vi "Add Numbers.vi"(8 "error in (no error)":errorcluster, 9 "Number 2":dbl, 10 "Number 1":dbl, 11 "Addition Actor in":refnum<class "Addition Actor.lvclass">) -> (0 "error out":errorcluster, 3 "Addition Actor out":refnum<class "Addition Actor.lvclass">)   [LabVIEW 2024, in "Addition Actor.lvclass"]
uses:
  Addition Actor.lvclass
  C:/Program Files/National Instruments/LabVIEW 2024/vi.lib/ActorFramework/Actor/Actor.lvclass
  <vilib>/ActorFramework/Actor/Actor.lvclass/Actor.ctl
  <vilib>/ActorFramework/Actor/Actor.lvclass
  Calculator Actor/Calculator Actor Messages/Addition Result Msg/Addition Result Msg.lvclass
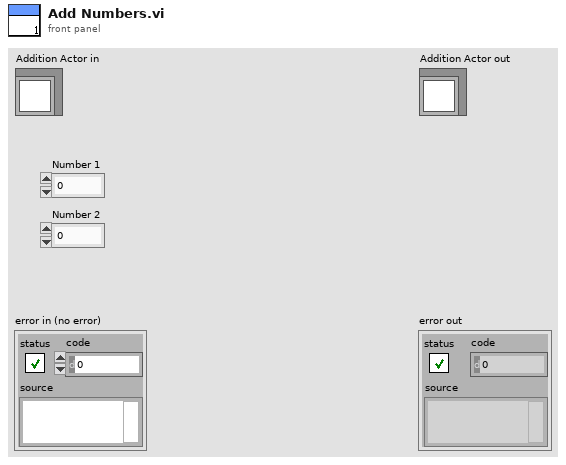
[diagram p1: front panel]
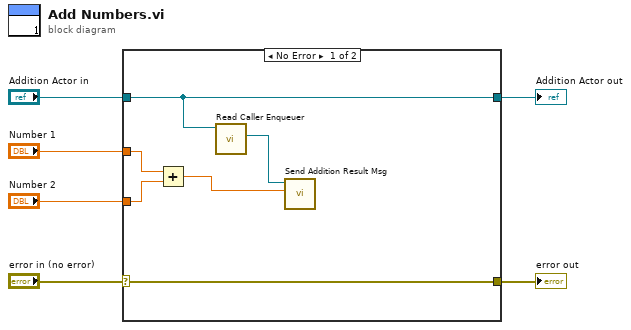
[diagram p0: block diagram]
diagram:
  n1 = case shown="No Error" "error in (no error)" {
    selector: "error in (no error)" -> [w12 w14]
    tunnel: [w12 w14] -> w5
    tunnel: [w9 w13] -> w3
    tunnel: "Addition Actor in" -> [w9 w13]
    tunnel: "Number 1" -> [w11 _]
    tunnel: "Number 2" -> [w10 _]
    frame No Error {
      n2 = Add(x=w11, y=w10) -> (x+y=w7:dbl)
      n3 = call <vilib>:"Read Caller Enqueuer.vi"("Actor"=w9) -> ("Caller Enqueuer"=w8:refnum<class "Message Enqueuer.lvclass">)  [unwired: 10 in]
      n4 = call "Send Addition Result Msg.vi"("Addition Result"=w7, "Message Enqueuer in"=w8) -> ()  [unwired: 8 in, 2 out]
    }
    frame Error {
    }
  }
  "error out" <- w5
  "Addition Actor out" <- w3
